vi "register_net_events_callback.vi"(6 "Events to register":T2[](array[typedef]), 8 "error in (no error)":errorcluster, 10 "NotifyIcon User Event Ref":T1, 11 "BalloonNotifier in":refnum<class "BalloonNotifier.lvclass">) -> (0 "error out":errorcluster, 2 ".NET event refs":refnum<k27>[](array[refnum]), 3 "BalloonNotifier out":refnum<class "BalloonNotifier.lvclass">)   [LabVIEW 2010, in "BalloonNotifier.lvclass"]
uses:
  BalloonNotifier.lvclass
  balloon_events.ctl
  ballloon_user_event_ref.ctl
  balloon_NET_Callback_Parameter.ctl
  BalloonNotifier.lvclass/BalloonNotifier.ctl
  balloon_event_data.ctl
  System.Windows.Forms
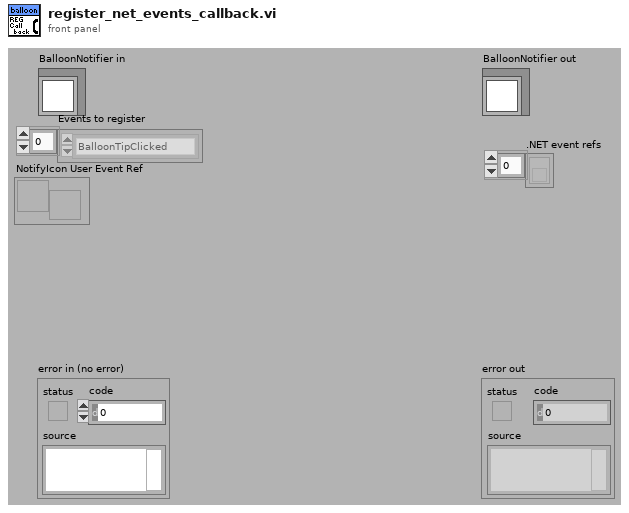
[diagram p1: front panel]
types:
  T1 = typedef "BalloonNotifier.lvclass/ballloon_user_event_ref.ctl" = refnum<user-event>
  T2 = typedef "BalloonNotifier.lvclass/balloon_events.ctl" = enum16{"BalloonTipClicked", "BalloonTipClosed", "BalloonTipShown", "Click", "Disposed", "DoubleClick", "MouseClick", "MouseDoubleClick", "MouseDown", "MouseMove", "MouseUp", "MenuItemClick", "MenuItemSelect"}
  T3 = typedef "BalloonNotifier.lvclass/balloon_NET_callback_parameter.ctl" = cluster{"NotifyIcon User Event Ref":T1, "Event Data":variant}
  T4 = typedef "BalloonNotifier.lvclass/balloon_event_data.ctl" = cluster{"NotifyIcon Event":T2, "Data String":string}
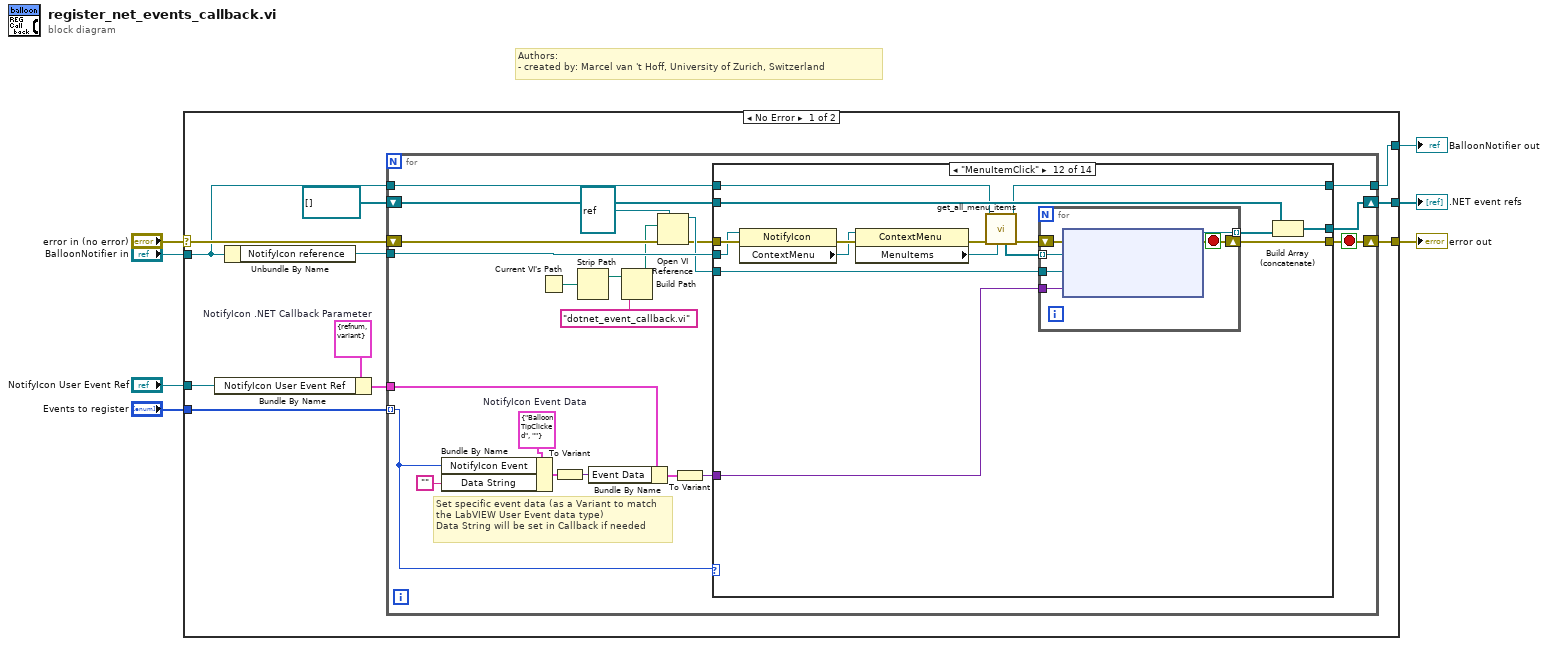
[diagram p0: block diagram]
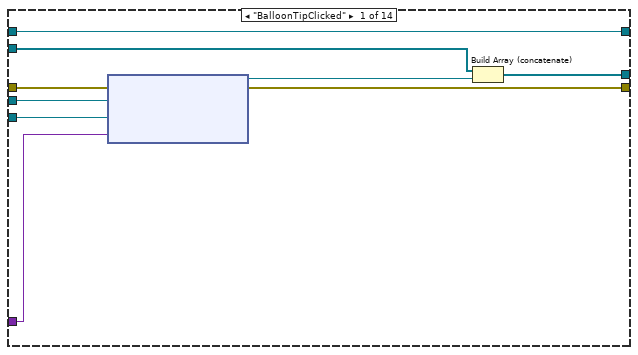
[diagram p2: hidden frame]
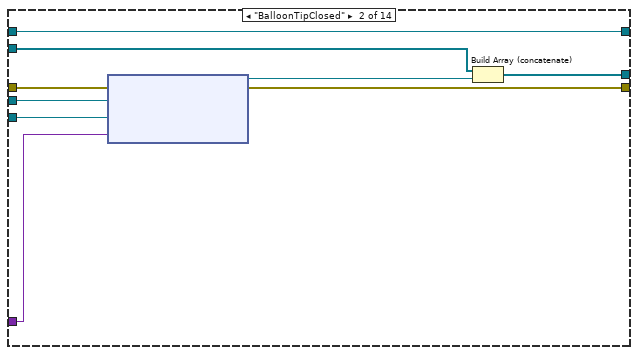
[diagram p3: hidden frame]
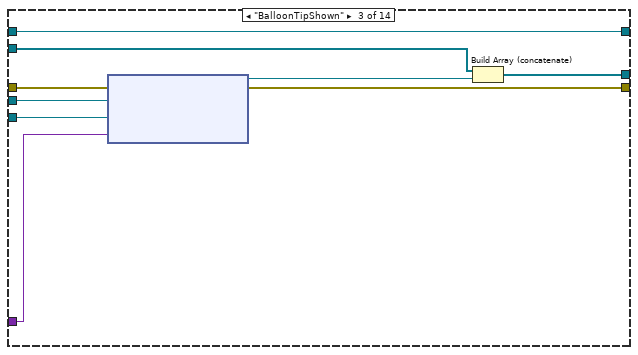
[diagram p4: hidden frame]
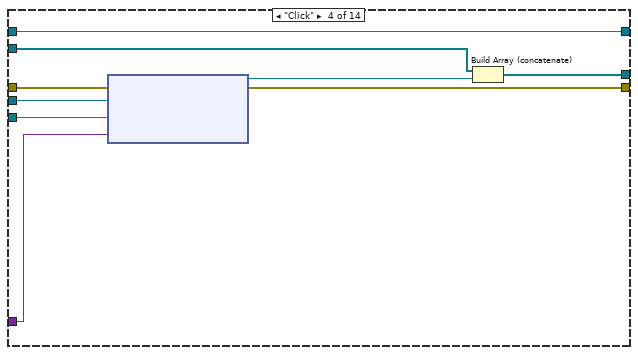
[diagram p5: hidden frame]
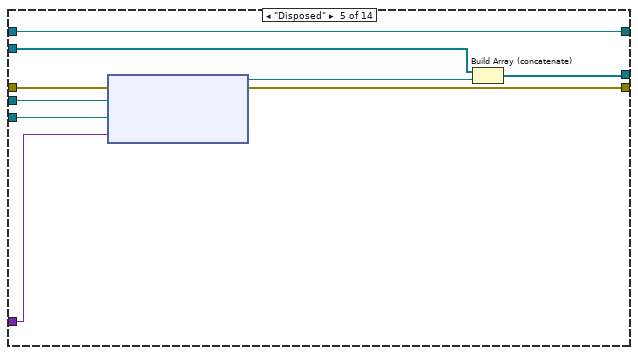
[diagram p6: hidden frame]
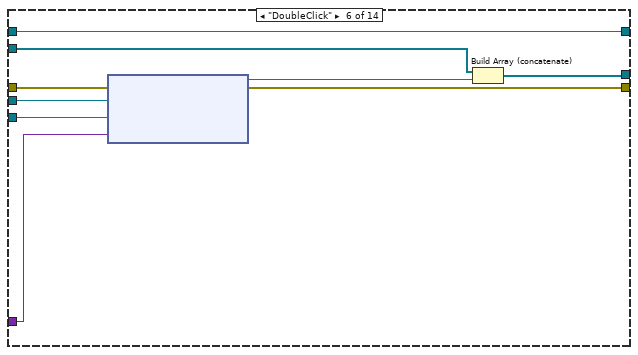
[diagram p7: hidden frame]
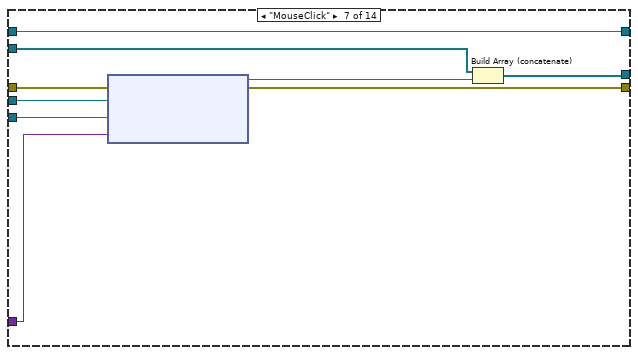
[diagram p8: hidden frame]
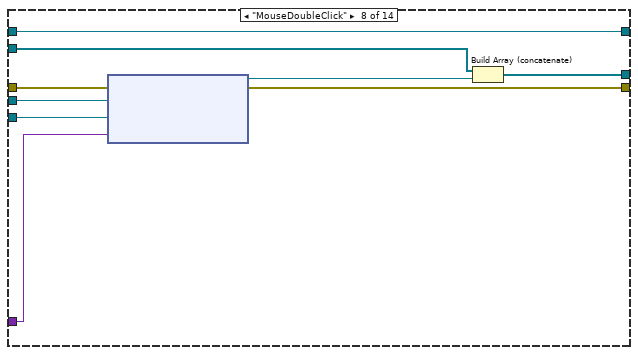
[diagram p9: hidden frame]
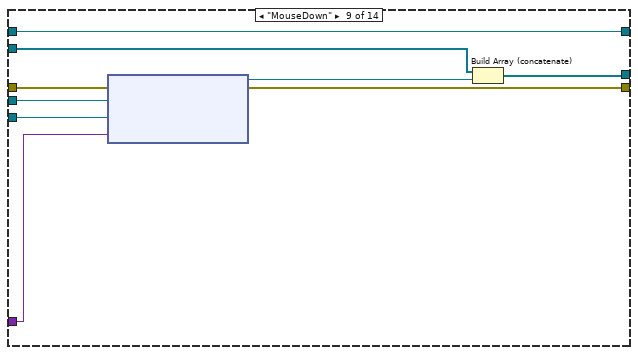
[diagram p10: hidden frame]
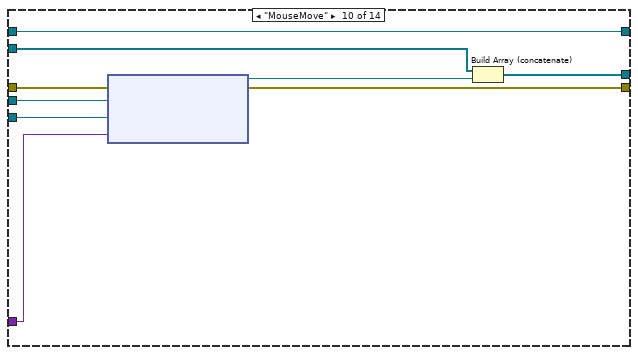
[diagram p11: hidden frame]
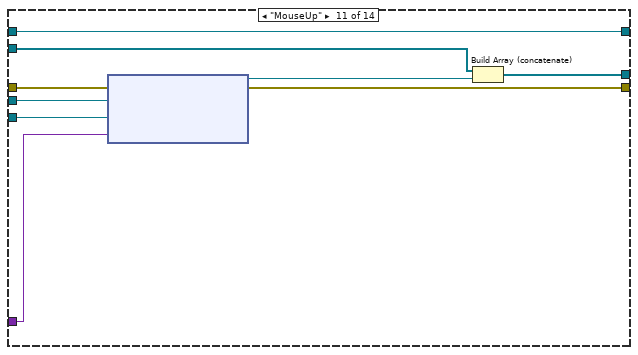
[diagram p12: hidden frame]
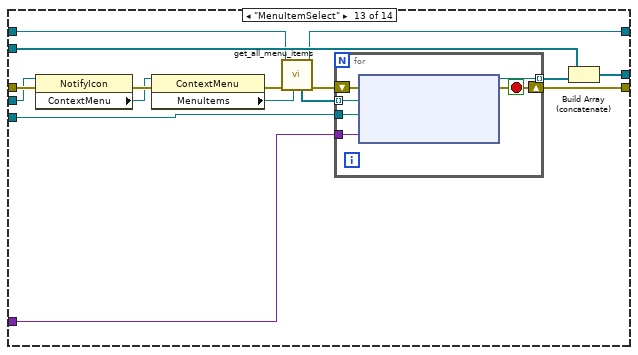
[diagram p13: hidden frame]
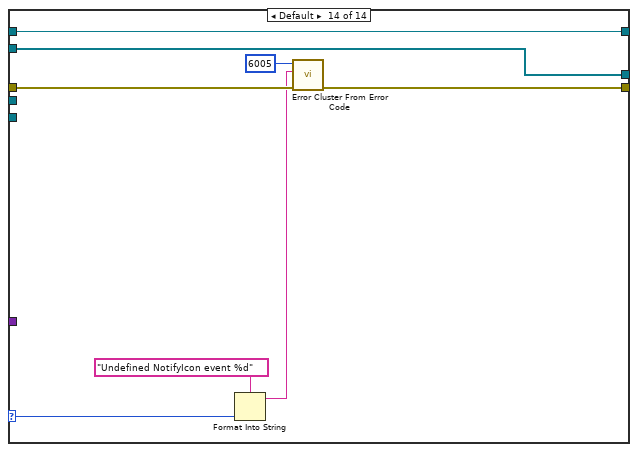
[diagram p14: hidden frame]
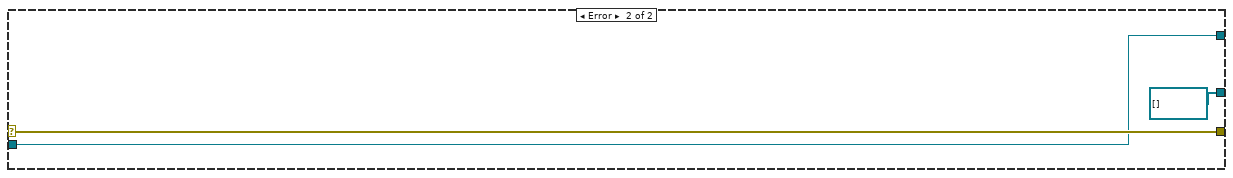
[diagram p15: hidden frame]
diagram:
  # "Authors: \n- created by: Marcel van 't Hoff, University of Zurich, Switzerland"
  n1 = case shown="No Error" "error in (no error)" {
    selector: "error in (no error)" -> [w11 w194]
    tunnel: "NotifyIcon User Event Ref" -> [w17 _]
    tunnel: "Events to register" -> [w16 _]
    tunnel: [w14 w194] -> w6
    tunnel: [w12 refnum<k27>[] []] -> w1
    tunnel: "BalloonNotifier in" -> [w9 w192]
    tunnel: [w8 w192] -> w2
    frame No Error {
      w18 = T3 {"NotifyIcon User Event Ref"=refnum, "Event Data"=variant}  # NotifyIcon .NET Callback Parameter
      n2 = Bundle By Name(cluster=w18, "NotifyIcon User Event Ref"=w17) -> (w15:T3)
      n3 = Unbundle By Name(w9) -> ("NotifyIcon reference"=w10:refnum<k24>)
      n4 = for {
        tunnel: w10 -> [w40]
        tunnel: w16 -> [w30] mode=indexing
        tunnel: w15 -> [w36]
        shift-right: [w29] -> w14
        shift-left: w11 -> [w24]
        shift-right: [w33] -> w12
        shift-left: refnum<k27>[] [] -> [w32]
        tunnel: w9 -> [w28]
        tunnel: [w27] -> w8
        stop <- w29 stop-if-true
        w39 = T4 {"NotifyIcon Event"=enum."BalloonTipClicked", "Data String"=""}  # NotifyIcon Event Data
        # "Set specific event data (as a Variant to match\nthe LabVIEW User Event data type)\nData String will be set in Callback if needed"
        n5 = Bundle By Name(cluster=w39, "NotifyIcon Event"=w30, "Data String"="") -> (w38:T4)
        n6 = Current VI's Path() -> (path=w22:path)
        n7 = To Variant(anything=w38) -> (Variant=w37:variant)
        n8 = Strip Path(path=w22) -> (stripped path=w21:path)  [unwired: 1 out]
        n9 = Bundle By Name(cluster=w36, "Event Data"=w37) -> (w35:T3)
        n10 = Build Path(base path=w21, name or relative path="dotnet_event_callback.vi") -> (appended path=w19:path)
        n11 = Open VI Reference(type specifier VI Refnum (for type only)=refnum<vi> refnum, vi path=w19, error in (no error)=w24) -> (vi reference=w25:refnum<vi>, error out=w23:errorcluster)  [unwired: 3 in]
        n12 = To Variant(anything=w35) -> (Variant=w34:variant)
        n13 = case shown="\"MenuItemClick\"" w30 {
          selector: w30 -> [_ _ _ _ _ _ _ _ _ _ _ _ _ w185]
          tunnel: w25 -> [w49 w58 w67 w76 w85 w94 w103 w112 w121 w130 w139 w140 w162 _]
          tunnel: w40 -> [w48 w57 w66 w75 w84 w93 w102 w111 w120 w129 w138 w152 w174 _]
          tunnel: w23 -> [w47 w56 w65 w74 w83 w92 w101 w110 w119 w128 w137 w153 w175 w189]
          tunnel: [w46 w55 w64 w73 w82 w91 w100 w109 w118 w127 w136 w150 w172 w190] -> w29
          tunnel: w34 -> [w45 w54 w63 w72 w81 w90 w99 w108 w117 w126 w135 w151 w173 _]
          tunnel: [w43 w52 w61 w70 w79 w88 w97 w106 w115 w124 w133 w149 w171 w191] -> w33
          tunnel: w32 -> [w42 w51 w60 w69 w78 w87 w96 w105 w114 w123 w132 w148 w169 w191]
          tunnel: w28 -> [w41 w50 w59 w68 w77 w86 w95 w104 w113 w122 w131 w146 w164 w184]
          tunnel: [w41 w50 w59 w68 w77 w86 w95 w104 w113 w122 w131 w145 w163 w184] -> w27
          frame "BalloonTipClicked" {
            n14 = node(w47, w48, w49, w45) -> (w44:refnum<k27>, w46:errorcluster)  [unwired: 1 in]
            n15 = Build Array (concatenate)(w42, w44) -> (w43:refnum<k27>[])
          }
          frame "BalloonTipClosed" {
            n16 = node(w56, w57, w58, w54) -> (w53:refnum<k27>, w55:errorcluster)  [unwired: 1 in]
            n17 = Build Array (concatenate)(w51, w53) -> (w52:refnum<k27>[])
          }
          frame "BalloonTipShown" {
            n18 = node(w65, w66, w67, w63) -> (w62:refnum<k27>, w64:errorcluster)  [unwired: 1 in]
            n19 = Build Array (concatenate)(w60, w62) -> (w61:refnum<k27>[])
          }
          frame "Click" {
            n20 = node(w74, w75, w76, w72) -> (w71:refnum<k27>, w73:errorcluster)  [unwired: 1 in]
            n21 = Build Array (concatenate)(w69, w71) -> (w70:refnum<k27>[])
          }
          frame "Disposed" {
            n22 = node(w83, w84, w85, w81) -> (w80:refnum<k27>, w82:errorcluster)  [unwired: 1 in]
            n23 = Build Array (concatenate)(w78, w80) -> (w79:refnum<k27>[])
          }
          frame "DoubleClick" {
            n24 = node(w92, w93, w94, w90) -> (w89:refnum<k27>, w91:errorcluster)  [unwired: 1 in]
            n25 = Build Array (concatenate)(w87, w89) -> (w88:refnum<k27>[])
          }
          frame "MouseClick" {
            n26 = node(w101, w102, w103, w99) -> (w98:refnum<k27>, w100:errorcluster)  [unwired: 1 in]
            n27 = Build Array (concatenate)(w96, w98) -> (w97:refnum<k27>[])
          }
          frame "MouseDoubleClick" {
            n28 = node(w110, w111, w112, w108) -> (w107:refnum<k27>, w109:errorcluster)  [unwired: 1 in]
            n29 = Build Array (concatenate)(w105, w107) -> (w106:refnum<k27>[])
          }
          frame "MouseDown" {
            n30 = node(w119, w120, w121, w117) -> (w116:refnum<k27>, w118:errorcluster)  [unwired: 1 in]
            n31 = Build Array (concatenate)(w114, w116) -> (w115:refnum<k27>[])
          }
          frame "MouseMove" {
            n32 = node(w128, w129, w130, w126) -> (w125:refnum<k27>, w127:errorcluster)  [unwired: 1 in]
            n33 = Build Array (concatenate)(w123, w125) -> (w124:refnum<k27>[])
          }
          frame "MouseUp" {
            n34 = node(w137, w138, w139, w135) -> (w134:refnum<k27>, w136:errorcluster)  [unwired: 1 in]
            n35 = Build Array (concatenate)(w132, w134) -> (w133:refnum<k27>[])
          }
          frame "MenuItemClick" {
            n36 = property class="NotifyIcon"(reference=w152, error in=w153) -> (error out=w155:errorcluster, "ContextMenu"=w154:refnum<k24>)  [unwired: 1 out]
            n37 = property class="ContextMenu"(reference=w154, error in=w155) -> (error out=w144:errorcluster, "MenuItems"=w143:refnum<k24>)  [unwired: 1 out]
            n38 = call-dynamic "get_all_menu_items.vi"("MenuItem Collection reference"=w143, "error in (no error)"=w144, "BalloonNotifier in"=w146) -> ("error out"=w141:errorcluster, "BalloonNotifier out"=w145:refnum<class "BalloonNotifier.lvclass">, "MenuItem references out"=w142:refnum<k24>[])  [unwired: 6 in]
            n39 = for {
              tunnel: w142 -> [w160] mode=indexing
              tunnel: w140 -> [w156]
              tunnel: w151 -> [w159]
              shift-right: [w157] -> w150
              shift-left: w141 -> [w161]
              tunnel: [w158] -> w147 mode=indexing
              stop <- w157 stop-if-true
              n40 = node(w161, w160, w156, w159) -> (w158:refnum<k27>, w157:errorcluster)  [unwired: 1 in]
            }
            n41 = Build Array (concatenate)(w148, w147) -> (w149:refnum<k27>[])
          }
          frame "MenuItemSelect" {
            n42 = property class="NotifyIcon"(reference=w174, error in=w175) -> (error out=w177:errorcluster, "ContextMenu"=w176:refnum<k24>)  [unwired: 1 out]
            n43 = property class="ContextMenu"(reference=w176, error in=w177) -> (error out=w167:errorcluster, "MenuItems"=w168:refnum<k24>)  [unwired: 1 out]
            n44 = call-dynamic "get_all_menu_items.vi"("MenuItem Collection reference"=w168, "error in (no error)"=w167, "BalloonNotifier in"=w164) -> ("error out"=w165:errorcluster, "BalloonNotifier out"=w163:refnum<class "BalloonNotifier.lvclass">, "MenuItem references out"=w166:refnum<k24>[])  [unwired: 6 in]
            n45 = for {
              tunnel: w166 -> [w182] mode=indexing
              tunnel: w162 -> [w178]
              tunnel: w173 -> [w181]
              shift-right: [w179] -> w172
              shift-left: w165 -> [w183]
              tunnel: [w180] -> w170 mode=indexing
              stop <- w179 stop-if-true
              n46 = node(w183, w182, w178, w181) -> (w180:refnum<k27>, w179:errorcluster)  [unwired: 1 in]
            }
            n47 = Build Array (concatenate)(w169, w170) -> (w171:refnum<k27>[])
          }
          frame Default {
            n48 = Format Into String(format string="Undefined NotifyIcon event %d", w185) -> (resulting string=w187:string)  [unwired: 2 in, 1 out]
            n49 = call <vilib>:"Error Cluster From Error Code.vi"("error in (no error)"=w189, "error message (\"\")"=w187, "error code (0)"=6005) -> ("error out"=w190:errorcluster)  [unwired: 6 in]
          }
        }
      }
    }
    frame Error {
    }
  }
  "error out" <- w6
  "BalloonNotifier out" <- w2
  ".NET event refs" <- w1
